vi "initializer_init_panel.vi"(0 "File Cluster":refnum<vi>, 1 "Starttime":refnum<vi>, 2 "Endtime":refnum<vi>, 7 "Run Button":refnum<vi>, 11 "Parameters Tree":refnum<vi>) -> ()   [LabVIEW 2019]
uses:
  lib/libSpecValiReader/libSpecValiReader.lvlib
panel:
  # "*******************************************************************\nBiogas Plant Control\n\nAuthor: Paul Zügel\nGCSC-Frankfurt am Main 2020\n\n*******************************************************************"
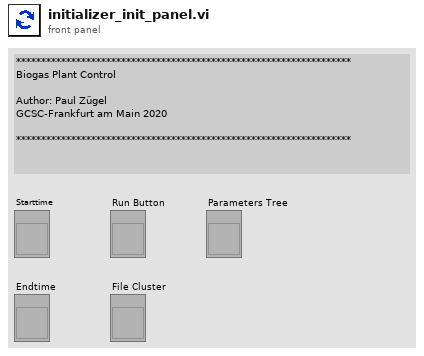
[diagram p1: front panel]
types:
  T1 = cluster{"Sim File Loaded":refnum<vi>, "Vali File Loaded":refnum<vi>, "Spec File Loaded":refnum<vi>}
  T2 = enum8{"Enabled", "Disabled", "Disabled and Grayed Out"}
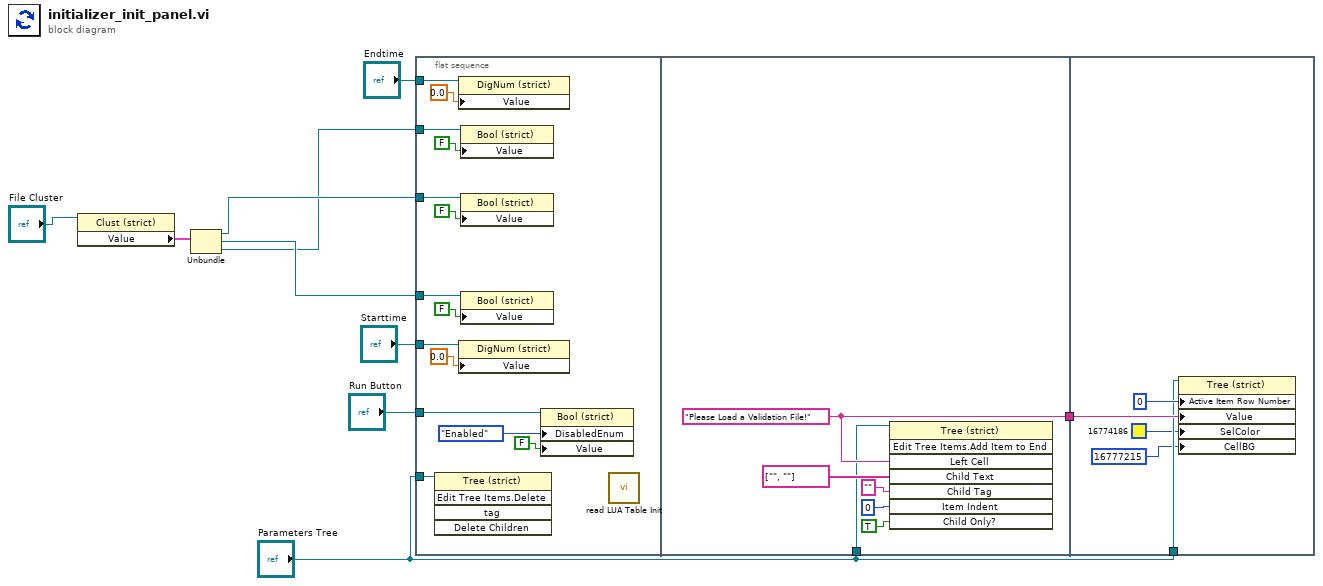
[diagram p0: block diagram]
diagram:
  n1 = property class="Clust (strict)"(reference="File Cluster") -> ("Value"=w4:T1)  [unwired: 1 in, 2 out]
  n2 = Unbundle(w4) -> ("Sim File Loaded"=w3:refnum<vi>, "Vali File Loaded"=w2:refnum<vi>, "Spec File Loaded"=w1:refnum<vi>)
  n3 = flat-sequence {
    tunnel: w2 -> [w23]
    tunnel: "Parameters Tree" -> [w22]
    tunnel: w1 -> [w21]
    tunnel: w3 -> [w18]
    tunnel: "Starttime" -> [w17]
    tunnel: "Endtime" -> [w16]
    tunnel: "Run Button" -> [w13]
    tunnel: [w27] -> w10
    tunnel: "Parameters Tree" -> [w25]
    tunnel: w10 -> [w34]
    tunnel: "Parameters Tree" -> [w33]
    frame #0 {
      n4 = invoke on="Invoke Node" class="Tree (strict)" method="Edit Tree Items.Delete"(reference=w22) -> ()  [unwired: 4 in, 5 out]
      n5 = property class="DigNum (strict)"(reference=w16, "Value"=0.0) -> ()  [unwired: 1 in, 2 out]
      n6 = property class="DigNum (strict)"(reference=w17, "Value"=0.0) -> ()  [unwired: 1 in, 2 out]
      n7 = property class="Bool (strict)"(reference=w21, "Value"=FALSE) -> ()  [unwired: 1 in, 2 out]
      n8 = property class="Bool (strict)"(reference=w18, "Value"=FALSE) -> ()  [unwired: 1 in, 2 out]
      n9 = property class="Bool (strict)"(reference=w23, "Value"=FALSE ("Vali File Loaded")) -> ()  [unwired: 1 in, 2 out]
      n10 = property class="Bool (strict)"(reference=w13, "DisabledEnum"=T2."Enabled" ("Disabled"), "Value"=FALSE ("Blinking")) -> ()  [unwired: 1 in, 2 out]
      n11 = call "read LUA Table Init.vi"() -> ()  [unwired: 11 in, 1 out]
    }
    frame #1 {
      w27 = "Please Load a Validation File!" ("Parent Tag")
      n12 = invoke on="Invoke Node" class="Tree (strict)" method="Edit Tree Items.Add Item to End"(reference=w25, "Left Cell"=w27, "Child Text"=string[] ["", ""], "Child Tag"="", "Item Indent"=0 ("New Item Indentation"), "Child Only?"=TRUE) -> ()  [unwired: 2 in, 8 out]
    }
    frame #2 {
      n13 = property on="Property Node" class="Tree (strict)"(reference=w33, "Active Item Row Number"=0 ("Active Item:Row Number"), "Value"=w34, "SelColor"=u32 16774186, "CellBG"=u32 16777215 ("Active Cell:Background Color")) -> ()  [unwired: 1 in, 2 out]
    }
  }
